vi "2 Ball 1114.vi"(1 "Run?":bool) -> (0 "Done?":bool)   [LabVIEW 2013]
uses:
  Globals/Homes.vi
  Globals/Useful Values.vi
panel:
  out "Time Elapsed":dbl
  out "Sum":dbl
  out "Ready for Vision?":bool
  out "Side":dbl
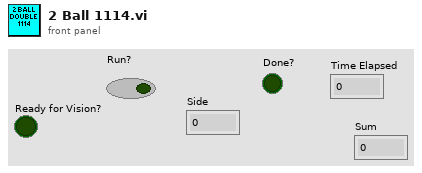
[diagram p1: front panel]
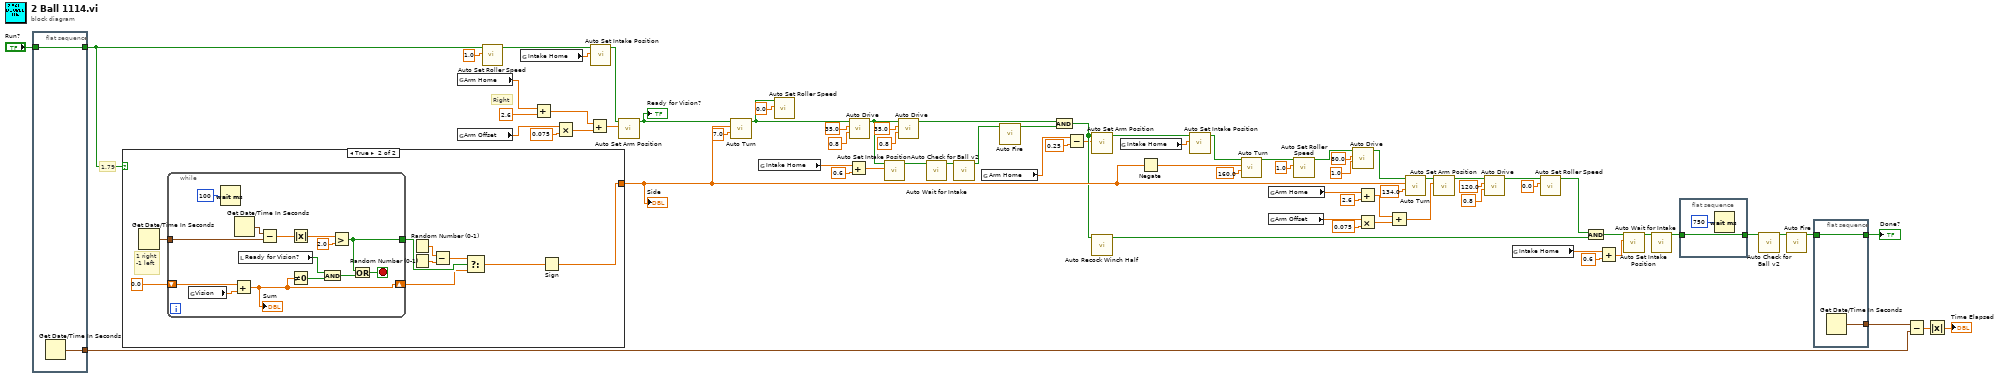
[diagram p0: block diagram]
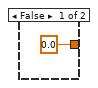
[diagram p2: hidden frame]
diagram:
  # "Right"
  # "1.79"
  n1 = flat-sequence {
    tunnel: "Run?" -> [w78]
    tunnel: [w78] -> w66
    tunnel: [w77] -> w62
    frame #0 {
      n2 = Get Date/Time In Seconds() -> (seconds since 1Jan1904=w77:timestamp)
    }
  }
  n3 = case shown="True" w66 {
    tunnel: [0.0 w80] -> w57
    frame False {
    }
    frame True {
      # "1 right\n-1 left"
      n4 = Get Date/Time In Seconds() -> (seconds since 1Jan1904=w87:timestamp)
      n5 = while {
        shift-right: [w98] -> w82
        shift-left: 0.0 -> [w101]
        tunnel: w87 -> [w96]
        tunnel: [w89] -> w83
        stop <- w91 stop-if-true
        n6 = global read "Useful Values.vi" "Vision"() -> (w102:dbl)
        n7 = Wait (ms)(milliseconds to wait=u32 100) -> ()  [unwired: 1 out]
        n8 = Add(x=w101, y=w102) -> (x+y=w98:dbl)
        "Sum" <- w98
        n9 = Get Date/Time In Seconds() -> (seconds since 1Jan1904=w95:timestamp)
        n10 = local read "Ready for Vision?"() -> (w99:bool)
        n11 = Subtract(x=w95, y=w96) -> (x-y=w94:dbl)
        n12 = Absolute Value(x=w94) -> (abs(x)=w93:dbl)
        n13 = Not Equal To 0?(x=w98) -> (x != 0?=w97:bool)
        n14 = And(x=w99, y=w97) -> (x .and. y?=w90:bool)
        n15 = Greater?(x=w93, y=2.0) -> (0:w89:bool)
        n16 = Or(x=w89, y=w90) -> (x .or. y?=w91:bool)
      }
      n17 = Random Number (0-1)() -> (number: 0 to 1=w84:dbl)
      n18 = Random Number (0-1)() -> (number: 0 to 1=w85:dbl)
      n19 = Subtract(x=w84, y=w85) -> (x-y=w86:dbl)
      n20 = Select(t=w86, s=w83, f=w82) -> (s? t:f=w81:dbl)
      n21 = Sign(1:w81) -> (0:w80:dbl)
    }
  }
  "Side" <- w57
  n22 = global read "Homes.vi" "Arm Home"() -> (w75:dbl)
  n23 = global read "Useful Values.vi" "Arm Offset"() -> (w73:dbl)
  n24 = call "Auto Set Roller Speed.vi"("Value"=1.0, "Run?"=w66) -> ("Done"=w68:bool)  [unwired: 9 in]
  n25 = global read "Homes.vi" "Intake Home"() -> (w76:dbl)
  n26 = Add(x=w75, y=2.6) -> (x+y=w70:dbl)
  n27 = Multiply(x=w73, y=0.075) -> (x*y=w71:dbl)
  n28 = Add(x=w70, y=w71) -> (x+y=w60:dbl)
  n29 = call "Auto Set Intake Position.vi"("Intake Position"=w76, "Run?"=w68) -> ("Done"=w61:bool)  [unwired: 9 in]
  n30 = call "Auto Set Arm Position.vi"("Arm Position"=w60, "Run?"=w61) -> ("Done"=w3:bool)  [unwired: 9 in]
  "Ready for Vision?" <- w3
  n31 = call "Auto Turn.vi"("Turn Amount"=7.0, "+/-?"=w57, "Run?"=w3) -> ("Done"=w2:bool)  [unwired: 8 in]
  n32 = global read "Homes.vi" "Intake Home"() -> (w53:dbl)
  n33 = call "Auto Set Roller Speed.vi"("Value"=0.0, "Run?"=w2) -> ()  [unwired: 9 in, 1 out]
  n34 = Add(x=w53, y=0.6) -> (x+y=w51:dbl)
  n35 = call "Auto Drive.vi"("Speed"=0.8, "Amount"=35.0, "Run?"=w2) -> ("Done"=w10:bool)  [unwired: 8 in]
  n36 = call "Auto Set Intake Position.vi"("Intake Position"=w51, "Run?"=w10) -> ("Done"=w50:bool)  [unwired: 9 in]
  n37 = call "Auto Drive.vi"("Speed"=0.8, "Amount"=35.0, "Run?"=w10) -> ("Done"=w9:bool)  [unwired: 8 in]
  n38 = call "Auto Wait for Intake.vi"("Run?"=w50) -> ("Done"=w48:bool)  [unwired: 10 in]
  n39 = call "Auto Check for Ball v2.vi"("Run?"=w48) -> ("Done"=w47:bool)  [unwired: 10 in]
  n40 = global read "Homes.vi" "Arm Home"() -> (w40:dbl)
  n41 = call "Auto Fire.vi"("Run?"=w47) -> ("Done"=w49:bool)  [unwired: 10 in]
  n42 = And(x=w9, y=w49) -> (x .and. y?=w41:bool)
  n43 = Subtract(x=w40, y=0.25) -> (x-y=w38:dbl)
  n44 = call "Auto Set Arm Position.vi"("Arm Position"=w38, "Run?"=w41) -> ("Done"=w37:bool)  [unwired: 9 in]
  n45 = call "Auto Recock Winch Half.vi"("Run?"=w41) -> ("Done"=w20:bool)  [unwired: 10 in]
  n46 = global read "Homes.vi" "Intake Home"() -> (w35:dbl)
  n47 = Negate(x=w57) -> (-x=w8:dbl)
  n48 = call "Auto Set Intake Position.vi"("Intake Position"=w35, "Run?"=w37) -> ("Done"=w36:bool)  [unwired: 9 in]
  n49 = call "Auto Turn.vi"("Turn Amount"=160.0, "+/-?"=w8, "Run?"=w36) -> ("Done"=w43:bool)  [unwired: 8 in]
  n50 = global read "Homes.vi" "Arm Home"() -> (w27:dbl)
  n51 = global read "Useful Values.vi" "Arm Offset"() -> (w31:dbl)
  n52 = call "Auto Set Roller Speed.vi"("Value"=1.0, "Run?"=w43) -> ("Done"=w44:bool)  [unwired: 9 in]
  n53 = call "Auto Drive.vi"("Speed"=1.0, "Amount"=80.0, "Run?"=w44) -> ("Done"=w25:bool)  [unwired: 8 in]
  n54 = Add(x=w27, y=2.6) -> (x+y=w28:dbl)
  n55 = Multiply(x=w31, y=0.075) -> (x*y=w29:dbl)
  n56 = Add(x=w28, y=w29) -> (x+y=w26:dbl)
  n57 = call "Auto Turn.vi"("Turn Amount"=134.0, "+/-?"=w57, "Run?"=w25) -> ("Done"=w24:bool)  [unwired: 8 in]
  n58 = call "Auto Set Arm Position.vi"("Arm Position"=w26, "Run?"=w24) -> ("Done"=w13:bool)  [unwired: 9 in]
  n59 = call "Auto Drive.vi"("Speed"=0.8, "Amount"=120.0, "Run?"=w13) -> ("Done"=w1:bool)  [unwired: 8 in]
  n60 = global read "Homes.vi" "Intake Home"() -> (w16:dbl)
  n61 = call "Auto Set Roller Speed.vi"("Value"=0.0, "Run?"=w1) -> ("Done"=w14:bool)  [unwired: 9 in]
  n62 = And(x=w14, y=w20) -> (x .and. y?=w7:bool)
  n63 = Add(x=w16, y=0.6) -> (x+y=w18:dbl)
  n64 = call "Auto Set Intake Position.vi"("Intake Position"=w18, "Run?"=w7) -> ("Done"=w19:bool)  [unwired: 9 in]
  n65 = call "Auto Wait for Intake.vi"("Run?"=w19) -> ("Done"=w6:bool)  [unwired: 10 in]
  n66 = flat-sequence {
    tunnel: w6 -> [w104]
    tunnel: [w104] -> w5
    frame #0 {
      n67 = Wait (ms)(milliseconds to wait=u32 750) -> ()  [unwired: 1 out]
    }
  }
  n68 = call "Auto Check for Ball v2.vi"("Run?"=w5) -> ("Done"=w21:bool)  [unwired: 10 in]
  n69 = call "Auto Fire.vi"("Run?"=w21) -> ("Done"=w59:bool)  [unwired: 10 in]
  n70 = flat-sequence {
    tunnel: [w106] -> w65
    tunnel: [w105] -> w58
    tunnel: w59 -> [w105]
    frame #0 {
      n71 = Get Date/Time In Seconds() -> (seconds since 1Jan1904=w106:timestamp)
    }
  }
  n72 = Subtract(x=w65, y=w62) -> (x-y=w64:dbl)
  n73 = Absolute Value(x=w64) -> (abs(x)=→"Time Elapsed":dbl)
  "Done?" <- w58
